vi "Read Auto Refresh.vi"(8 "error in (no error)":errorcluster, 10 "Config Data":T1, 11 "Connection Data In":T3) -> (0 "error out":errorcluster, 1 "Adquisition Data Out":T2, 3 "Connection Data Out":T3)   [LabVIEW 2014, in "MSX-E3711_dll.lvlib"]
doc: "Inicia la adquisición de datos en modo AutoRefresh. Al mismo tiempo lee el estado de las I/O."
uses:
  MSX-E3711_dll.lvlib
  Typedef/Connection Data.ctl
  E:/Repositorio Magnis/INF002/v0/Modules/HAL/Drivers/Sync/ADDI-DATA MSX-E3711/API/MSXE371x.dll
  MSXE371x.dll
  E:/Repositorio Magnis/INF002/v0/Modules/HAL/Drivers/Sync/ADDI-DATA MSX-E3711/API/MXCommon.dll
  MXCommon.dll
  Typedef/Adquisition Data.ctl
  Typedef/Config Data.ctl
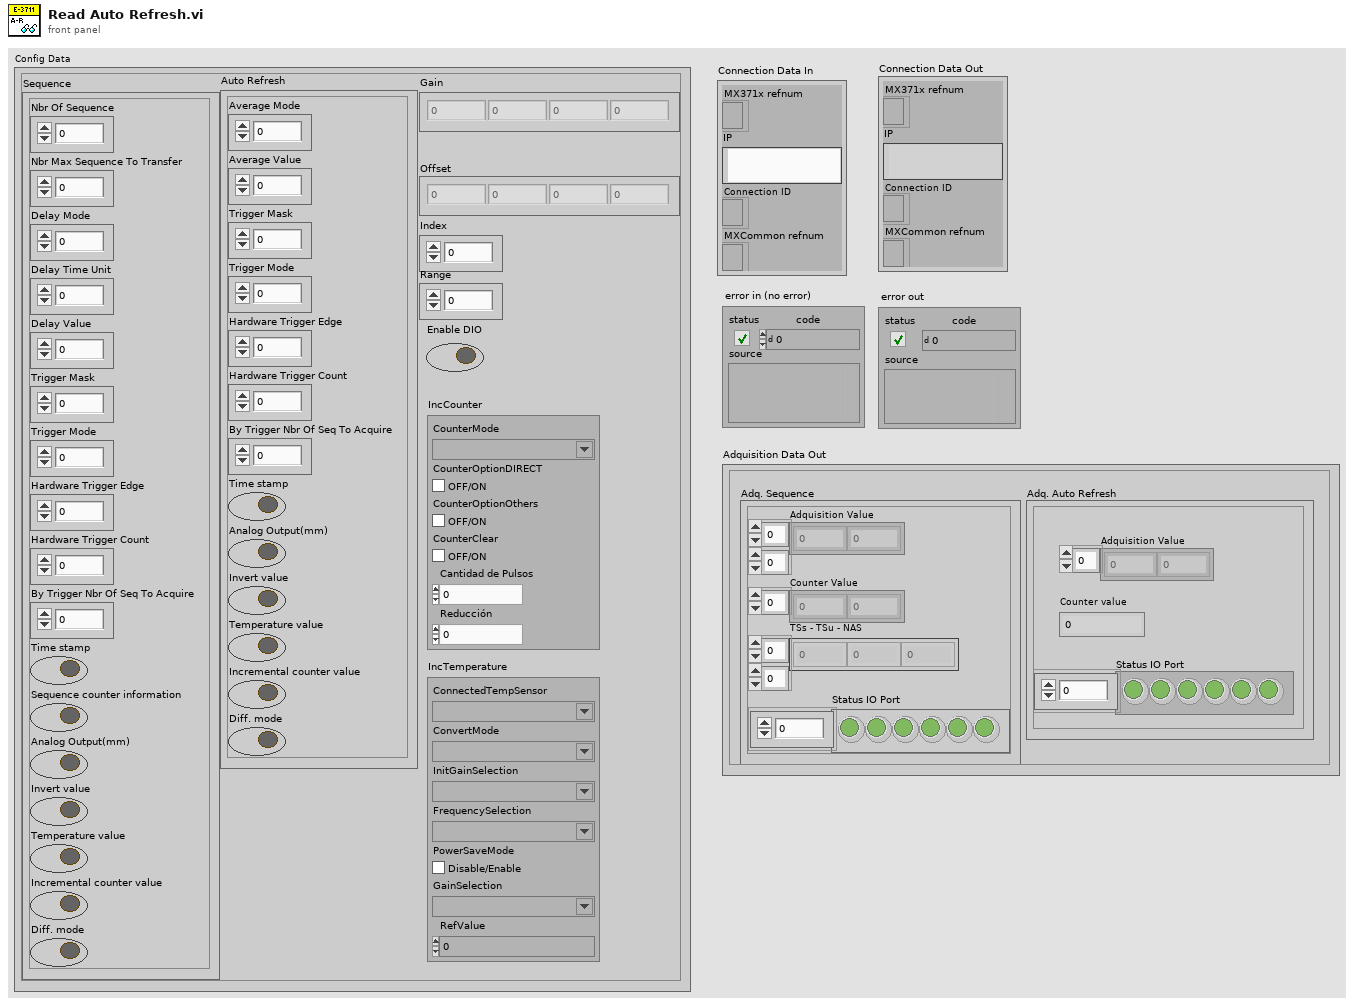
[diagram p1: front panel]
types:
  T1 = typedef "MSX-E3711_dll.lvlib/Config Data.ctl" = cluster{"Auto Refresh":cluster{"Average Mode":u64, "Average Value":u64, "Trigger Mask":u64, "Trigger Mode":u64, "Hardware Trigger Edge":u64, "Hardware Trigger Count":u64, "By Trigger Nbr Of Seq To Acquire":u64, "Time stamp":bool, "Analog Output(mm)":bool, "Invert value":bool, "Temperature value":bool, "Incremental counter value":bool, "Diff. mode":bool}, "Gain":sgl[], "Offset":sgl[], "Index":u64, "Range":sgl, "Sequence":cluster{"Nbr Of Sequence":u64, "Nbr Max Sequence To Transfer":u64, "Delay Mode":u64, "Delay Time Unit":u64, "Delay Value":u64, "Trigger Mask":u64, "Trigger Mode":u64, "Hardware Trigger Edge":u64, "Hardware Trigger Count":u64, "By Trigger Nbr Of Seq To Acquire":u64, "Time stamp":bool, "Sequence counter information":bool, "Analog Output(mm)":bool, "Invert value":bool, "Temperature value":bool, "Incremental counter value":bool, "Diff. mode":bool}, "Enable DIO":bool, "IncCounter":cluster{"CounterMode":string, "CounterOptionDIRECT  ":bool, "CounterOptionOthers":bool, "CounterClear ":bool, "Cantidad de Pulsos":sgl, "Reducción":sgl}, "IncTemperature":cluster{"ConnectedTempSensor":string, "ConvertMode":string, "InitGainSelection":string, "FrequencySelection":string, "PowerSaveMode":bool, "GainSelection":string, "RefValue":dbl}}
  T2 = typedef "MSX-E3711_dll.lvlib/Adquisition Data.ctl" = cluster{"Adq. Sequence":cluster{"Adquisition Value":u32[][], "Counter Value":u32[], "TSs - TSu - NAS":u64[][], "Status IO Port":bool[]}, "Adq. Auto Refresh":cluster{"Adquisition Value":u64[], "Status IO Port":bool[], "Counter value":u32}}
  T3 = typedef "MSX-E3711_dll.lvlib/Connection Data.ctl" = cluster{"MX371x refnum":refnum<k24>, "IP":string, "Connection ID ":refnum<k5>, "MXCommon refnum":refnum<k24>}
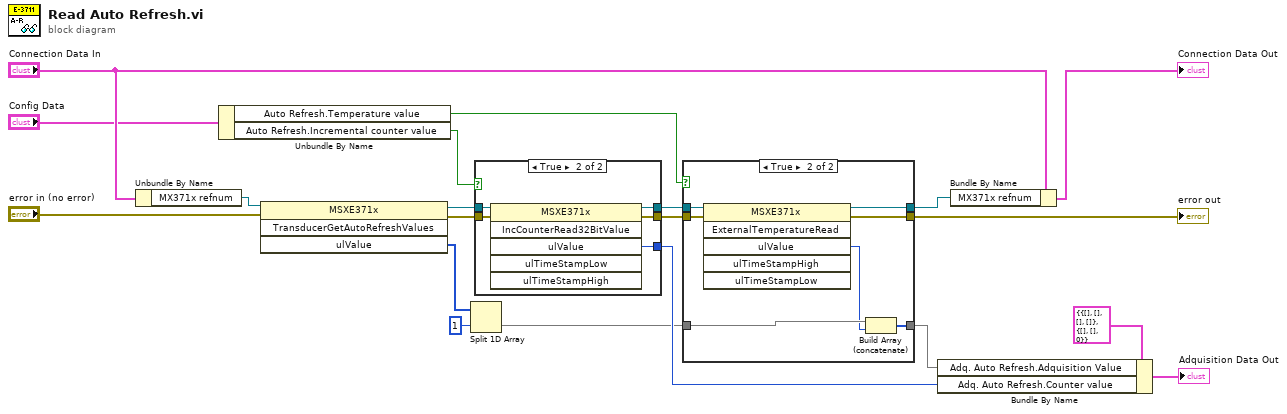
[diagram p0: block diagram]
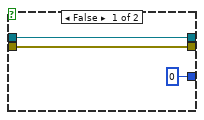
[diagram p3: hidden frame]
diagram:
  n1 = Unbundle By Name("Connection Data In") -> ("MX371x refnum"=w18:refnum<k24>)
  n2 = Unbundle By Name("Config Data") -> ("Auto Refresh.Temperature value"=w6:bool, "Auto Refresh.Incremental counter value"=w7:bool)
  n3 = invoke class="MSXE371x" method="TransducerGetAutoRefreshValues"(reference=w18, error in="error in (no error)") -> (reference out=w15:refnum<k24>, error out=w14:errorcluster, "ulValue"=w3:u64[])  [unwired: 2 in, 1 out]
  n4 = Split 1D Array(array=w3, index=1) -> (second subarray=w2:u64[])  [unwired: 1 out]
  n5 = case shown="True" w7 {
    tunnel: w15 -> [w23 w28]
    tunnel: w14 -> [w22 w27]
    tunnel: [w23 w26] -> w13
    tunnel: [w22 w25] -> w12
    tunnel: [u64 0 ("ulValue") w24] -> w5
    frame False {
    }
    frame True {
      n6 = invoke class="MSXE371x" method="IncCounterRead32BitValue"(reference=w28, error in=w27) -> (reference out=w26:refnum<k24>, error out=w25:errorcluster, "ulValue"=w24:u64)  [unwired: 4 in, 3 out]
    }
  }
  n7 = case shown="True" w6 {
    tunnel: w13 -> [w31 w38]
    tunnel: w12 -> [w30 w37]
    tunnel: [w31 w36] -> w11
    tunnel: [w30 w35] -> w10
    tunnel: w2 -> [w29 w34]
    tunnel: [w29 w32] -> w4
    frame False {
    }
    frame True {
      n8 = invoke class="MSXE371x" method="ExternalTemperatureRead"(reference=w38, error in=w37) -> (reference out=w36:refnum<k24>, error out=w35:errorcluster, "ulValue"=w33:u64)  [unwired: 4 in, 3 out]
      n9 = Build Array (concatenate)(w34, w33) -> (w32:u64[])
    }
  }
  "error out" <- w10
  n10 = Bundle By Name(cluster=T2 {"Adq. Sequence"={"Adquisition Value"=[], "Counter Value"=[], "TSs - TSu - NAS"=[], "Status IO Port"=[]}, "Adq. Auto Refresh"={"Adquisition Value"=[], "Status IO Port"=[], "Counter value"=0}} ("Adquisition Data Out 2"), "Adq. Auto Refresh.Adquisition Value"=w4, "Adq. Auto Refresh.Counter value"=w5) -> (→"Adquisition Data Out":T2)
  n11 = Bundle By Name(cluster="Connection Data In", "MX371x refnum"=w11) -> (→"Connection Data Out":T3)
